vi "create_configuration.vi"(8 "error in (no error)":errorcluster, 10 "pixels_array_in":u8[][](array[numeric]), 11 "configuration input":string="{\n \t\"actor_id\": \"\",\n \"lights\": [\n    { \"array_id\": \"LightArray_0\",\n    \"coneLights\": [\n        { \n         \"attach_socket\": \"\",\n         \"attenuation_radius\": 10000.0,\n         \"backlight_attenuation_radius\": 20.0,\n         \"backlight_color\": {\n          \"a\": 1,\n          \"b\": 1,\n          \"g\": 1,\n          \"r\": 1\n         },\n         \"backlight_indirect_lighting_intensity\": 10.0,\n         \"backlight_intensity\": 20.0,\n         \"backlight_location\": {\n          \"x\": 100.0,\n          \"y\": 10.0,\n          \"z\":10.0\n         },\n         \"backlight_soft_source_radius\": 2.0,\n         \"backlight_source_length\": 1.0,\n         \"backlight_source_radius\": 1.0,\n         \"backlight_temperature\": 8000.0,\n         \"backlight_volumetric_scattering_intensity\": 10.0,\n         \"color\": {\n          \"a\": 1,\n          \"b\": 1,\n          \"g\": 1,\n          \"r\": 1\n         },\n         \"description\": \"\",\n         \"enable_backlight\": true,\n         \"enable_directional_light\": true,\n         \"enable_streaming\": true,\n         \"ies_profile\": \"None\",\n         \"indirect_lighting_intensity\": 1.0,\n         \"inner_cone_angle\": 8.0,\n         \"intensity\": 200000.0,\n         \"led\": 0,\n         \"light_function\": \"\",\n\t\t \"listen_port\": 0,\n         \"location\": {\n          \"x\": 233.0,\n          \"y\": 71.0,\n          \"z\": 84.0\n         },\n         \"outer_cone_angle\": 16.0,\n         \"parent_component_attachment\": \"\",\n         \"raytrace_global_ilum\": false,\n         \"raytrace_reflection\": false,\n         \"raytrace_shadow\": false,\n         \"receive_stream\": true,\n         \"rotation\": {\n          \"pitch\": 0.0,\n          \"roll\": 0.0,\n          \"yaw\": 0.0\n         },\n         \"soft_source_radius\": 0.0,\n         \"source_length\": 1.0,\n         \"source_radius\": 0.0,\n         \"temperature\": 8000.0,\n         \"type\": \"None\",\n         \"use_attach_socket\": true,\n         \"use_light_function\": true,\n         \"use_parent_component_attachment\": false,\n         \"volumetric_scattering_intensity\": 5.0,\n         \"wait_for_fresh_frame\": true,\n         \"xres\": 200,\n         \"yres\": 100\n        }\n       ]\n    }],\n \"location\": {\n  \"x\": 0.0,\n  \"y\": 0.0,\n  \"z\": 0.0\n },\n \"rectLights\": [],\n \"rotation\": {\n  \"pitch\": 0.0,\n  \"roll\": 0.0,\n  \"yaw\": 0.0\n }\n}\n") -> (0 "error out":errorcluster, 3 "configuration output":string)   [LabVIEW 2019, in "Lib_Simx.lvlib"]
doc: "Converting array of pixels to JSON string."
uses:
  Lib_Simx.lvlib
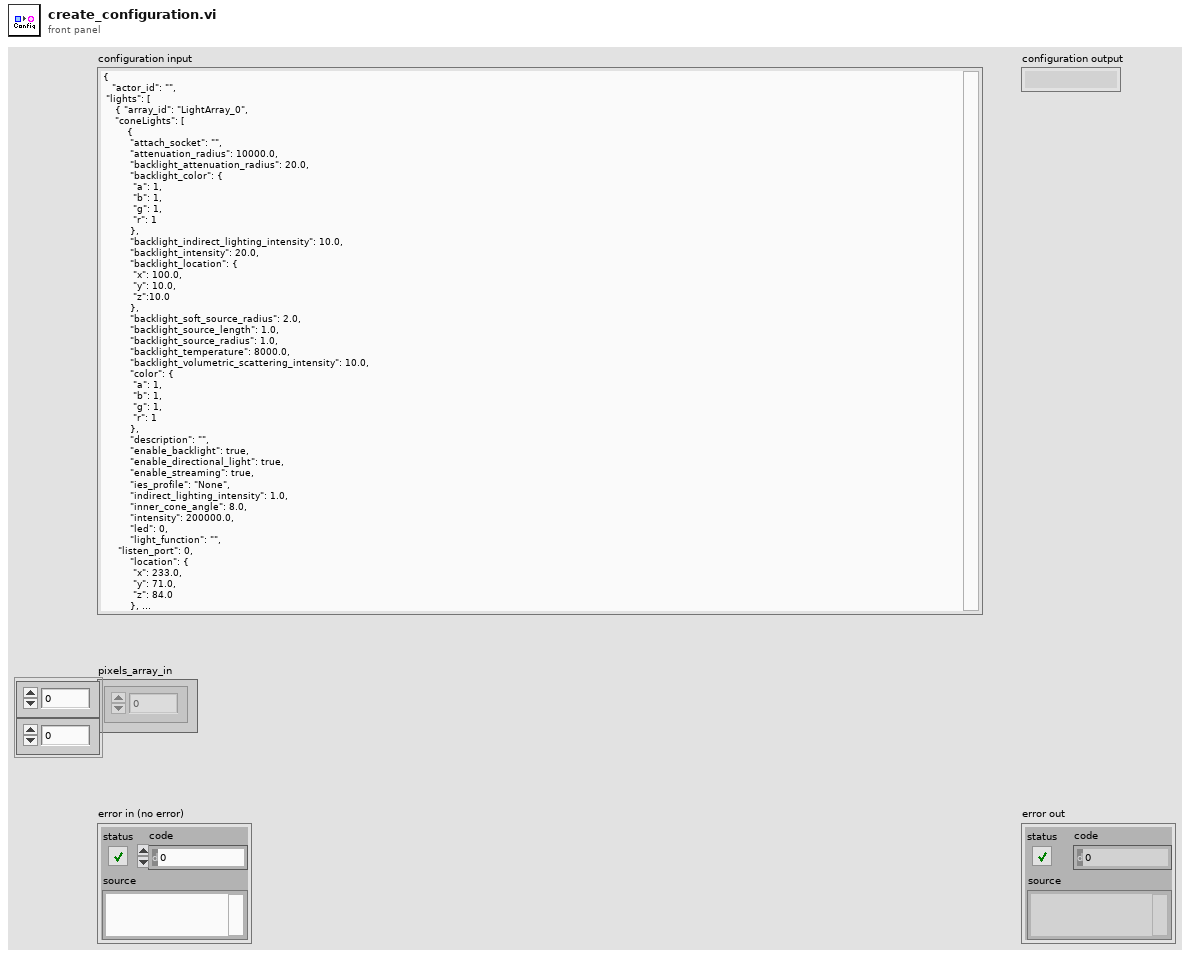
[diagram p1: front panel]
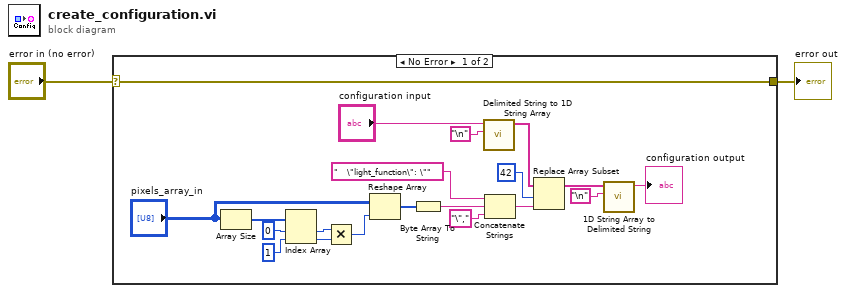
[diagram p0: block diagram]
diagram:
  n1 = case shown="No Error" "error in (no error)" {
    selector: "error in (no error)" -> [w12 w23]
    tunnel: [w12 w23] -> w1
    frame No Error {
      n2 = Array Size(array="pixels_array_in") -> (size(s)=w10:i32[])
      n3 = Index Array(array=w10, index #1=0 ("index"), index #2=1 ("index")) -> (element #1=w7:i32, element #2=w6:i32)
      n4 = Multiply(x=w7, y=w6) -> (x*y=w5:i32)
      n5 = Reshape Array("pixels_array_in", w5) -> (w4:u8[])
      n6 = Byte Array To String(unsigned byte array=w4) -> (string=w3:string)
      n7 = call <vilib>:"Delimited String to 1D String Array.vi"("delimiter"="\n", "delimited string"="configuration input") -> ("string array"=w14:string[])  [unwired: 9 in]
      n8 = Concatenate Strings("   \"light_function\": \"", w3, "\",") -> (w15:string)
      n9 = Replace Array Subset(array=w14, new element=w15, index=42) -> (w17:string[])
      n10 = call <vilib>:"1D String Array to Delimited String.vi"("delimiter"="\n", "string array"=w17) -> ("delimited string"=→"configuration output":string)  [unwired: 9 in]
    }
    frame Error {
    }
  }
  "error out" <- w1
